vi "Lian_Lab04_I.vi"() -> ()   [LabVIEW 2020]
uses:
  <vilib>/express/express analysis/Spectral/Block/exnSpectralBlock spectral measurements peak poly.vi
  <vilib>/express/express analysis/Spectral/Block/exnSpectralBlock spectral measurements peak DDT.vi
  <vilib>/express/express analysis/Spectral/XNode/ExpressSpectralMeasurementsBlockNode.xnode
panel:
  in  "?":bool
  out "Waveform Chart":dynamicdata(graph)
  out "Waveform Graph":dynamicdata(graph)
  in  "Rate":dbl=1000.0
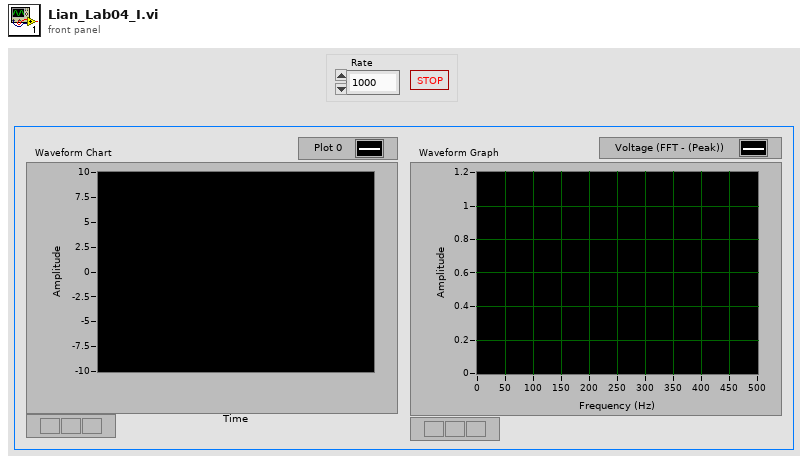
[diagram p1: front panel]
types:
  T1 = cluster{"averaging mode":u16, "weighting mode":u16, "number of averages":u32}
  T2 = cluster{"dB On (F)":bool, "unwrap phase (F)":bool, "convert to degree (F)":bool}
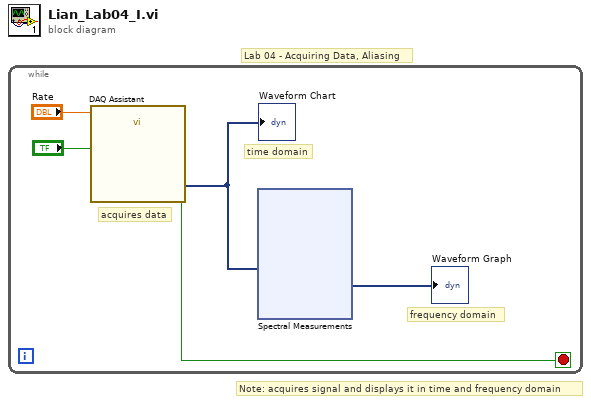
[diagram p0: block diagram]
diagram:
  # "Lab 04 - Acquiring Data, Aliasing"
  # "Note: acquires signal and displays it in time and frequency domain"
  n1 = while {
    stop <- w5 stop-if-true
    # "acquires data"
    # "frequency domain"
    # "time domain"
    n2 = call "DAQ Assistant"("rate"="Rate", "stop (F)"="?") -> ("data"=w2:dynamicdata, "stopped"=w5:bool)  [unwired: 14 in, 2 out]
    "Waveform Chart" <- w2
    n3 = xnode "Spectral Measurements"("Signals"=w2) -> ("FFT - (Peak)"=→"Waveform Graph":dynamicdata)  [unwired: 1 in, 2 out]
  }
